vi "Test Class translation.vi"() -> ()   [LabVIEW 2012]
uses:
  CRDS Class/Data Class/Main Class/CRDS Data.lvclass
  Reusable/CRDS/Data/Main/CRDS Data.lvclass
panel:
  out "ClassName":string
  out "NameLen":u32
  out "substring":string
  out "PStrLen":u32
  out "NumLevels":u32
  out "String":string
  out "length":i32
  out "data string":string
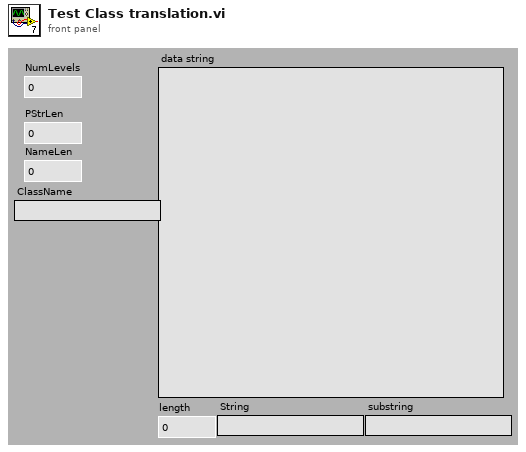
[diagram p1: front panel]
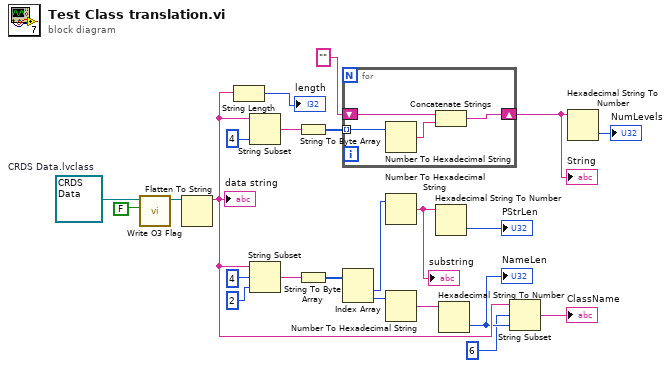
[diagram p0: block diagram]
diagram:
  w7 = refnum<class "CRDS Data.lvclass"> refnum  # CRDS Data.lvclass
  n1 = call "Write O3 Flag.vi"("O3 Flag"=FALSE, "CRDS Data in"=w7) -> ("CRDS Data out"=w5:refnum<class "CRDS Data.lvclass">)  [unwired: 8 in, 1 out]
  n2 = Flatten To String(anything=w5) -> (data string=w4:string)  [unwired: 3 in, 2 out]
  "data string" <- w4
  n3 = String Length(string=w4) -> (length=→"length":i32)
  n4 = String Subset(string=w4, length (rest)=4 ("length (rest)")) -> (substring=w15:string)  [unwired: 1 in]
  n5 = String Subset(string=w4, offset (0)=4 ("offset"), length (rest)=2 ("length (rest)")) -> (substring=w13:string)
  n6 = String To Byte Array(string=w15) -> (unsigned byte array=w20:u8[])
  n7 = String To Byte Array(string=w13) -> (unsigned byte array=w12:u8[])
  n8 = for {
    tunnel: w20 -> [w27] mode=indexing
    shift-right: [w24] -> w18
    shift-left: "" -> [w26]
    n9 = Number To Hexadecimal String(2:w27) -> (0:w25:string)  [unwired: 1 in]
    n10 = Concatenate Strings(w26, w25) -> (w24:string)
  }
  "String" <- w18
  n11 = Index Array(array=w12) -> (element #1=w11:u8, element #2=w9:u8)  [unwired: 2 in]
  n12 = Number To Hexadecimal String(2:w11) -> (0:w10:string)  [unwired: 1 in]
  "substring" <- w10
  n13 = Number To Hexadecimal String(2:w9) -> (0:w8:string)  [unwired: 1 in]
  n14 = Hexadecimal String To Number(string=w10) -> (number=→"PStrLen":u32)  [unwired: 2 in, 1 out]
  n15 = Hexadecimal String To Number(string=w8) -> (number=w3:u32)  [unwired: 2 in, 1 out]
  "NameLen" <- w3
  n16 = String Subset(string=w4, offset (0)=6, length (rest)=w3) -> (substring=→"ClassName":string)
  n17 = Hexadecimal String To Number(string=w18) -> (number=→"NumLevels":u32)  [unwired: 2 in, 1 out]
